vi "p2.vi"() -> ()   [LabVIEW 2021, in "d20.lvlib"]
uses:
  d20.lvlib
  Circular Buffer/Circular Buffer.lvclass
  AOC/AOC.lvlib
panel:
  out "mix":i32
  out "index":i32
  out "Answer":i64
  in  "Example":string="1\n2\n-3\n3\n-2\n0\n4"
  in  "Example":bool=TRUE
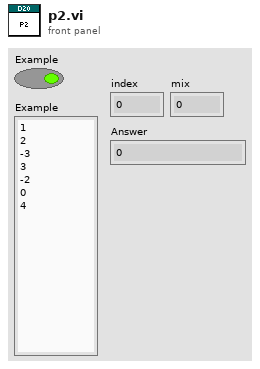
[diagram p1: front panel]
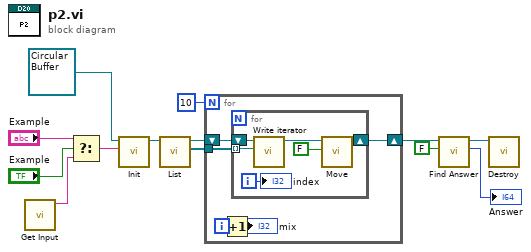
[diagram p0: block diagram]
diagram:
  n1 = call "Get Input.vi"() -> ("Input"=w13:string)  [unwired: 11 in]
  n2 = Select(t="Example", s="Example", f=w13) -> (s? t:f=w6:string)
  n3 = call "Init.vi"("Input"=w6, "Circular Buffer in"=refnum<class "Circular Buffer.lvclass"> refnum) -> ("Circular Buffer out"=w1:refnum<class "Circular Buffer.lvclass">)  [unwired: 9 in]
  n4 = call "List.vi"("Circular Buffer in"=w1) -> ("Node List"=w9:refnum<data-value>[], "Circular Buffer out"=w10:refnum<class "Circular Buffer.lvclass">)  [unwired: 7 in, 2 out]
  n5 = for {
    N: 10 -> [_]
    tunnel: w9 -> [w16]
    shift-right: [w17] -> w3
    shift-left: w10 -> [w18]
    i -> [w15]
    n6 = Increment(x=w15) -> (x+1=→"mix":i32)
    n7 = for {
      tunnel: w16 -> [w22] mode=indexing
      shift-right: [w21] -> w17
      shift-left: w18 -> [w23]
      i -> [w20]
      n8 = call "Write iterator.vi"("iterator"=w22, "Circular Buffer in"=w23) -> ("Circular Buffer out"=w24:refnum<class "Circular Buffer.lvclass">)  [unwired: 9 in]
      n9 = call "Move.vi"("P1"=FALSE, "Circular Buffer in"=w24) -> ("Circular Buffer out"=w21:refnum<class "Circular Buffer.lvclass">)  [unwired: 9 in]
      "index" <- w20
    }
  }
  n10 = call "Find Answer.vi"("P1"=FALSE, "Circular Buffer in"=w3) -> ("Answer"=→"Answer":i64, "Circular Buffer out"=w7:refnum<class "Circular Buffer.lvclass">)  [unwired: 8 in]
  n11 = call "Destroy.vi"("Circular Buffer in"=w7) -> ()  [unwired: 11 in]
